vi "Q8381 Query Wave Data to Array.vi"(5 "VISA resource name":refnum<visa-resource-name>, 6 "GPIB address":u16=8 step=1) -> (1 "X Axis Data":dbl[](array[numeric]) format="%.5e", 2 "Data Number":u16, 3 "GPIB status":bool, 4 "Y Axis Data":dbl[](array[numeric]) format="%.5e")   [LabVIEW 2017]
panel:
  out "Y Receive Data":string
  out "X Receive Data":string
  # "Change wave data to array"
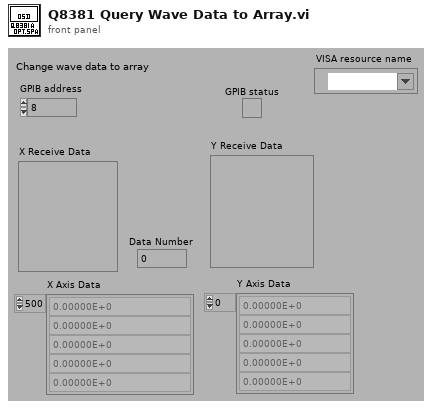
[diagram p1: front panel]
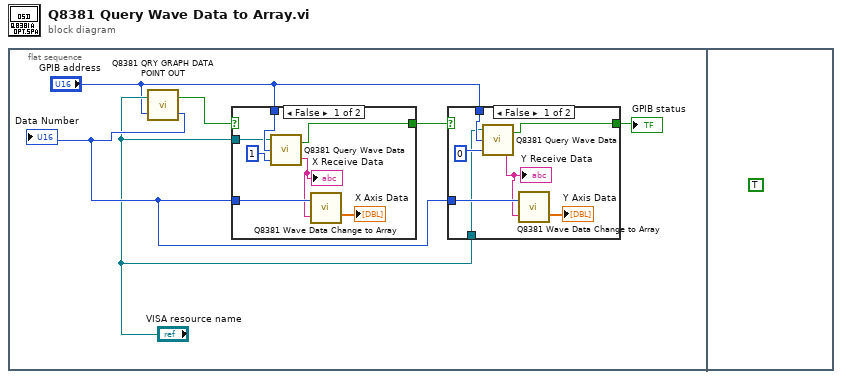
[diagram p0: block diagram]
diagram:
  n1 = flat-sequence {
    frame #0 {
      n2 = call "Q8381 QRY GRAPH DATA POINT OUT.vi"("GPIB address"="GPIB address", "VISA resource name"="VISA resource name") -> ("Data point"=w4:u16, "GPIB status"=w3:bool)
      "Data Number" <- w4
      n3 = case shown="False" w3 {
        selector: w3 -> [_ w22]
        tunnel: [w16 w22] -> w6
        tunnel: "GPIB address" -> [w19 _]
        tunnel: w4 -> [w20 _]
        tunnel: "VISA resource name" -> [w17 _]
        frame False {
          n4 = call "Q8381 Query Wave Data.vi"("set:"=1, "GPIB address"=w19, "VISA resource name"=w17) -> ("Received Data"=w15:string, "GPIB status"=w16:bool)
          "X Receive Data" <- w15
          n5 = call "Q8381 Wave Data Change to Array.vi"("Receive Data"=w15, "Data Number"=w20) -> ("Data Array"=→"X Axis Data":dbl[])
        }
        frame True {
        }
      }
      n6 = case shown="False" w6 {
        selector: w6 -> [_ w14]
        tunnel: "GPIB address" -> [w10 _]
        tunnel: [w7 w14] -> w5
        tunnel: w4 -> [w12 _]
        tunnel: "VISA resource name" -> [w9 _]
        frame False {
          n7 = call "Q8381 Query Wave Data.vi"("set:"=0, "GPIB address"=w10, "VISA resource name"=w9) -> ("Received Data"=w8:string, "GPIB status"=w7:bool)
          "Y Receive Data" <- w8
          n8 = call "Q8381 Wave Data Change to Array.vi"("Receive Data"=w8, "Data Number"=w12) -> ("Data Array"=→"Y Axis Data":dbl[])
        }
        frame True {
        }
      }
      "GPIB status" <- w5
    }
    frame #1 {
      (unwired) TRUE
    }
  }
